vi "Elevator Loop.vi"() -> ()   [LabVIEW 2017]
uses:
  <vilib>/Rock Robotics/WPI/ThirdParty/Phoenix-LabVIEW/Motor Controller/Controls/CTRE_Phoenix_MotorControl_ControlMode.ctl
  <vilib>/Rock Robotics/WPI/ThirdParty/Sensors/navX/_TypeDefs/FRIC_navX_DeviceNumbersTypeDef.ctl
  Robot Global Data.vi
  <vilib>/Rock Robotics/WPI/Solenoid/Deprecated/WPI_SolenoidSetBool.vi
panel:
  out "Reverse Limit Closed?":bool
  out "Forward Limit Closed?":bool
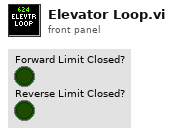
[diagram p1: front panel]
types:
  T1 = typedef "FRIC_navX_DeviceNumbersTypeDef.ctl" = enum16{"Dev0", "Dev1", "Dev2", "Dev3"}
  T2 = typedef "CTRE_Phoenix_MotorControl_ControlMode.ctl" = u16
  T3 = typedef "Dashboard Control Data.ctl" = cluster{"Drivetrain Settings Cluster":T4, "Intake Presets":T6, "Elevator Settings Cluster":T7, "Drivetrain Encoder Values":T9, "Auton Chooser":T10, "Auton Presets":cluster{"Start Position":dbl}, "Elevator Encoder Values":T11, "Pressure M":dbl, "Pressure B":dbl, "Zero All?":bool, "Enable Vision":bool}
  T4 = typedef "Drivetrain Settings Cluster.ctl" = cluster{"Gyro Steer PID Gains":T5, "Distance Drive PID Gains":T5, "Drive Tolerance":dbl, "Gyro Tolerance":dbl, "Gyro Output":dbl, "Distance Output":dbl, "Y Power Multiplier":dbl, "Turn Power Multiplier":dbl, "Creep Rate":dbl, "Encoder Reset":bool, "DT Mode Modifier":enum16{"None, Default", "Cube", "Square"}, "Left Encoder Tick Constant":dbl, "Right Encoder Tick Constant":dbl, "Shift Speed":dbl, "Zero Gyro":bool, "Y min":dbl, "Y max":dbl, "X min":dbl, "X max":dbl, "Finish Velocity":dbl, "Anti-tip peRcEnT":dbl}
  T5 = typedef "PID Gains Cluster.ctl" = cluster{"Proportional Gain":dbl, "Integral Time":dbl, "Derivative Time":dbl}
  T6 = typedef "Intake Presets.ctl" = cluster{"Idle Angle":dbl, "Mid Angle":dbl, "Low Angle":dbl, "Outtake Power":dbl, "Intake Power":dbl, "Unstuck":dbl, "Angle Tolerance":dbl, "Max Angle":dbl, "Max Current":dbl, "Current Trip Time":dbl, "Reset Encoder?":bool, "Encoder Scale":dbl, "PID gains":cluster{"proportional gain (Kc)":dbl, "integral time (Ti, min)":dbl, "derivative time (Td, min)":dbl}, "output range":cluster{"output high":dbl, "output low":dbl}, "IR Constant Pull Rate":dbl}
  T7 = typedef "Elevator Settings Cluster.ctl" = cluster{"Ground Height":dbl, "Switch Height":dbl, "Scale High Height ":dbl, "Scale Low Height":dbl, "Elevator PID Gains":T8, "Elevator Tolerance":dbl, "Reset Encoders":bool, "Encoder Scale":dbl, "Max Height":dbl, "Mid Height":dbl, "output range":cluster{"output high":dbl, "output low":dbl}, "Slow Down Tolerance":dbl, "Tick Constant":dbl, "Tip Constant":dbl, "Slow Down Multiplier":dbl, "Almost Tip Constant":dbl, "Bottom Trip Offset":dbl}
  T8 = typedef "PID Gains.ctl" = cluster{"proportional gain (Kc)":dbl, "integral time (Ti, min)":dbl, "derivative time (Td, min)":dbl}
  T9 = typedef "DT Encoder Values.ctl" = cluster{"Left Encoder":cluster{"Distance":dbl, "Speed":dbl, "Tick":dbl}, "Right Encoder":cluster{"Distance":dbl, "Speed":dbl, "Tick":dbl}}
  T10 = typedef "Auton Chooser.ctl" = cluster{"Left":bool, "Center":bool, "Right":bool, "Scale":bool, "Both":bool, "Switch":bool, "Test":bool, "No Script":bool}
  T11 = typedef "Elevator Encoder Values.ctl" = cluster{"Encoder Values":cluster{"Distance":dbl, "Speed":dbl, "Tick":dbl}}
  T12 = typedef "Dashboard Status Data.ctl" = cluster{"Elevator Status Cluster":T13, "Drivetrain Status Cluster":T16, "Intake Status Cluster":T18, "Climb Status Cluster":T21, "Intake PDP Info":T22, "Auton Command Cluster":T23, "Pressure ":dbl, "Auton Field Index":i32, "Auton File Index":i32, "Auton Side Index":i32, "Auton Side":string, "Field Config":string, "Robot Info":T24, "Auton Queue Index ":i32, "IMU Pitch Zero":dbl, "IMU Roll Zero":dbl, "IMU Yaw Zero":dbl}
  T13 = typedef "Elevator Status Cluster.ctl" = cluster{"Finished":bool, "Elevator Power":dbl, "Elevator State":T14, "Elevator Mode":T15, "Elevator Height":dbl, "At Bottom?":bool, "At Top?":bool, "Scale high?":bool, "PID Output":dbl, "2nd Gear":bool}
  T14 = typedef "Elevator State.ctl" = enum16{"Idle", "Ground", "Mid", "Scale", "Switch"}
  T15 = typedef "Elevator Mode.ctl" = enum16{"Semi Auto", "Manual", "Auto"}
  T16 = typedef "Drivetrain Status Cluster.ctl" = cluster{"Throttle (Y)":dbl, "Steer (X)":dbl, "Drivetrain Mode":T17, "Brake?":bool, "Distance Drive Complete?":bool, "PID Drive Complete?":bool, "Creep Mode?":bool, "Gyro Steer Complete?":bool, "Gyro":dbl, "Heading Target":dbl, "Distance Target":dbl, "2nd Gear":bool, "Drivetrain Encoder Values":T9}
  T17 = typedef "Drivetrain Mode.ctl" = enum16{"Manual", "Gyro Steer", "PID Drive", "Distance Drive", "Autonomous"}
  T18 = typedef "Intake Status Cluster.ctl" = cluster{"Intake Mode":T19, "Intake States":T20, "Intake Current Angle":dbl, "Cube In Posession?":bool, "Intake Wrist Up?":bool, "Right Roller Power":dbl, "Angle Power":dbl, "Left Roller Power":dbl}
  T19 = typedef "Intake Mode.ctl" = enum16{"Auto", "Semi Auto", "Manual"}
  T20 = typedef "Intake States.ctl" = enum16{"Zero", "Override Angle", "Idle", "Drop Mid", "Drop Low", "Outtake", "Intake"}
  T21 = typedef "Climb Status Cluster.ctl" = cluster{"Climb":bool, "Time Remaining":dbl, "Button Pressed":bool}
  T22 = typedef "Intake PDP Info.ctl" = cluster{"Voltage Percent Output":dbl, "Output Voltage":dbl, "Bus Voltage":dbl, "Device ID":dbl, "Output Current":dbl, "Sensor Velocity":dbl, "Sensor Position":dbl, "Pulse Width Position":dbl, "Pulse Width Velocity":dbl, "Temperature":dbl, "Inverted?":bool}
  T23 = typedef "Auton Command Cluster.ctl" = cluster{"commandID":dbl, "headingTarget":dbl, "async":dbl, "elevatorCommand":dbl, "intakeMode":dbl, "maxTime":dbl, "ySpeed":dbl, "zeroGyro":dbl, "intakeCommand":dbl, "distanceTarget":dbl, "xSpeed":dbl, "elevatorMode":dbl, "scaleHigh":dbl, "rollerSpeed":dbl, "intakeAngle":dbl, "manualOpen":dbl, "secondGear":dbl, "elevatorPower":dbl, "waitFor":dbl, "overrideAngle":dbl}
  T24 = typedef "Robot Info.ctl" = cluster{"FMS":bool, "Switch and Scale Sides":string, "Event Name":string, "Alliance":T25, "Position":T26, "Match Number":u16, "Robot Mode":T27, "Match Time(s)":sgl}
  T25 = typedef "WPI_DriverStationAllianceInfo.ctl" = enum16{"Red", "Blue", "Invalid"}
  T26 = typedef "WPI_DriverStationPositionInfo.ctl" = enum16{"1", "2", "3"}
  T27 = typedef "WPI_DriverStationRobotMode2.ctl" = enum16{"Autonomous Disabled", "Autonomous Enabled", "Teleop Disabled", "Teleop Enabled", "Disconnected", "Finish", "Test Disabled", "Test Enabled", "Emergency Stopped"}
  T28 = typedef "Elevator Command Cluster.ctl" = cluster{"Elevator Mode":T15, "Elevator State":T14, "Manual Speed":dbl, "Reset Encoders":bool, "High?":bool, "Climb?":bool, "Gear 2?":bool}
  T29 = typedef "WPI_SolenoidDevRef.ctl" = cluster{"DevStatus":errorcluster, "Pneumatics Control Module":u8, "Forward Solenoid Channel":T30, "Reverse Solenoid Channel":T30}
  T30 = typedef "WPI_SolenoidChannel.ctl" = enum8{"Solenoid 0", "Solenoid 1", "Solenoid 2", "Solenoid 3", "Solenoid 4", "Solenoid 5", "Solenoid 6", "Solenoid 7", "Invalid"}
  T31 = cluster{"Yaw":dbl, "Roll":dbl, "Pitch":dbl, "Heading":dbl, "Fused Heading":dbl}
  T32 = typedef "WPI_SwitchDevRef.ctl" = cluster{"DevStatus":errorcluster, "DIO Channel":T33, "CntIndex":T34, "Normally Closed":bool}
  T33 = typedef "FPGA_DIOChannel.ctl" = enum8{"DIO 0", "DIO 1", "DIO 2", "DIO 3", "DIO 4", "DIO 5", "DIO 6", "DIO 7", "DIO 8", "DIO 9", "DIO MXP 0", "DIO MXP 1", "DIO MXP 2", "DIO MXP 3", "DIO MXP 4", "DIO MXP 5", "DIO MXP 6", "DIO MXP 7", "DIO MXP 8", "DIO MXP 9", "DIO MXP 10", "DIO MXP 11", "DIO MXP 12", "DIO MXP 13", "DIO MXP 14", "DIO MXP 15", "SPI Port CS1", "SPI Port CS2", "SPI Port CS3", "SPI Port MISO", "SPI Port MOSI", "Invalid"}
  T34 = typedef "FPGA_CounterCtrSystemIndex.ctl" = enum8{"Ctr 0", "Ctr 1", "Ctr 2", "Ctr 3", "Ctr 4", "Ctr 5", "Ctr 6", "Ctr 7", "Invalid"}
  T35 = typedef "WPI_MotorControlDeviceRef.ctl" = cluster{"DeviceStatus":errorcluster, "Type":T36, "PWM":cluster{"PWM Channel":T37, "DeadBand":T38}, "CAN":cluster{"Device Number":u8, "SetOutput VI Ref":variant, "GetOutput VI Ref":variant, "Enable VI Ref":variant, "Disable VI Ref":variant, "Data":variant}, "Invert":bool, "DIO PWM":cluster{"PWM \"Enable\" Channel":T37, "DIOChannel":T33, "PWM Rate":dbl}}
  T36 = typedef "WPI_MotorControlType.ctl" = enum16{"PWM", "CAN", "DIO PWM"}
  T37 = typedef "FPGA_DIOPWMChannel.ctl" = enum8{"PWM 0", "PWM 1", "PWM 2", "PWM 3", "PWM 4", "PWM 5", "PWM 6", "PWM 7", "PWM 8", "PWM 9", "PWM MXP 0", "PWM MXP 1", "PWM MXP 2", "PWM MXP 3", "PWM MXP 4", "PWM MXP 5", "PWM MXP 6", "PWM MXP 7", "PWM MXP 8", "PWM MXP 9", "Invalid"}
  T38 = typedef "WPI_PWMDeadband.ctl" = cluster{"Name":string, "maxPositivePwm":i32, "minPositivePwm":i32, "centerPwm":i32, "maxNegativePwm":i32, "minNegativePwm":i32, "angularRange":u16}
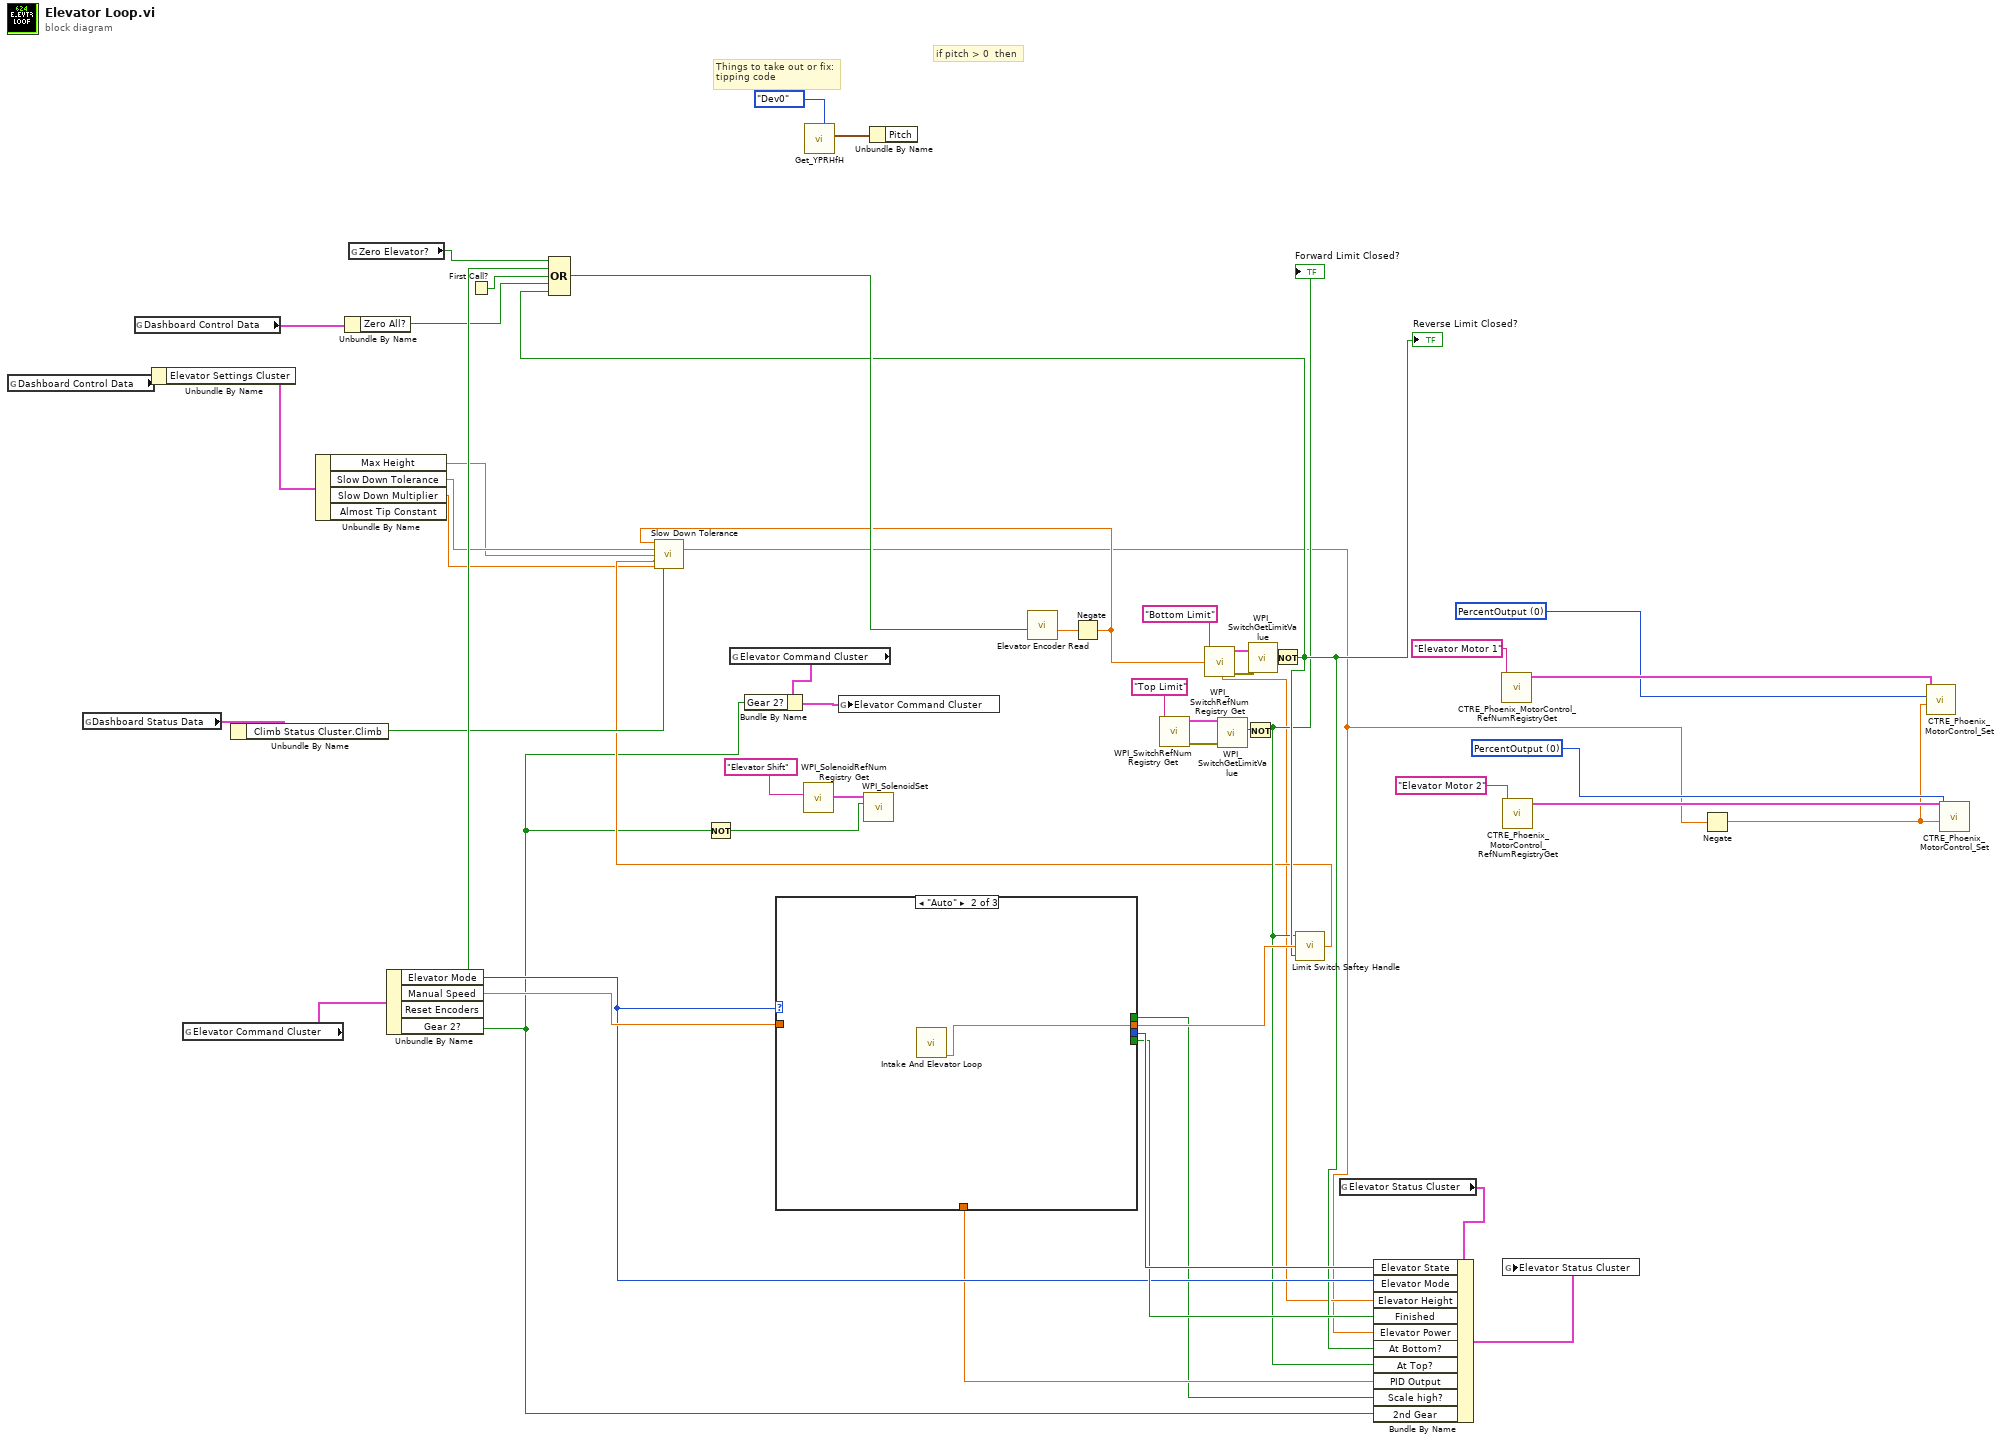
[diagram p0: block diagram]
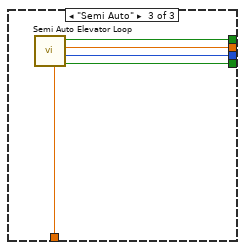
[diagram p3: hidden frame]
diagram:
  w37 = T2 0 items=["PercentOutput"=0, "Position"=1, "Velocity"=2, "Current"=3, "Follower"=5, "MotionProfile"=6, "MotionMagic"=7, "MotionMagicArc"=8, "MotionProfileArc"=10, "Disabled"=15] ("Control Mode")
  w36 = T2 0 items=["PercentOutput"=0, "Position"=1, "Velocity"=2, "Current"=3, "Follower"=5, "MotionProfile"=6, "MotionMagic"=7, "MotionMagicArc"=8, "MotionProfileArc"=10, "Disabled"=15] ("Control Mode")
  # "if pitch > 0  then"
  # "Things to take out or fix:\ntipping code"
  n1 = global read "Robot Global Data.vi" "Dashboard Control Data"() -> (w46:T3)
  n2 = global read "Robot Global Data.vi" "Dashboard Status Data"() -> (w31:T12)
  n3 = global read "Robot Global Data.vi" "Dashboard Control Data"() -> (w6:T3)
  n4 = Unbundle By Name(w46) -> ("Elevator Settings Cluster"=w45:T7)
  n5 = global read "Robot Global Data.vi" "Elevator Command Cluster"() -> (w42:T28)
  n6 = Unbundle By Name(w31) -> ("Climb Status Cluster.Climb"=w28:bool)
  n7 = Unbundle By Name(w45) -> ("Max Height"=w29:dbl, "Slow Down Tolerance"=w30:dbl, "Slow Down Multiplier"=w13:dbl)  [unwired: 1 out]
  n8 = Unbundle By Name(w6) -> ("Zero All?"=w5:bool)
  n9 = global read "Robot Global Data.vi" "Zero Elevator?"() -> (w44:bool)
  n10 = Unbundle By Name(w42) -> ("Elevator Mode"=w35:T15, "Manual Speed"=w41:dbl, "Reset Encoders"=w32:bool, "Gear 2?"=w1:bool)
  n11 = First Call?() -> (First Call?: T/F=w43:bool)
  n12 = Not(x=w1) -> (.not. x?=w2:bool)
  n13 = global read "Robot Global Data.vi" "Elevator Command Cluster"() -> (w11:T28)
  n14 = Bundle By Name(cluster=w11, "Gear 2?"=w1) -> (w12:T28)
  n15 = case shown="\"Auto\"" w35 {
    tunnel: [w53 w54 w59] -> w38
    tunnel: w41 -> [w53 _ _]
    tunnel: [_ _ w58] -> w40
    tunnel: [_ _ w57] -> w39
    tunnel: [_ _ w56] -> w33
    tunnel: [_ _ w55] -> w34
    frame "Manual", Default {
    }
    frame "Auto" {
      n16 = call "Intake And Elevator Loop.vi"() -> ("Elevator Power"=w54:dbl)  [unwired: 11 in, 4 out]
    }
    frame "Semi Auto" {
      n17 = call "Semi Auto Elevator Loop.vi"() -> ("Finished?"=w57:bool, "Elevator State"=w58:T14, "Elevator Power"=w59:dbl, "High?"=w56:bool, "PID Output"=w55:dbl)  [unwired: 7 in]
    }
  }
  n18 = call <vilib>:"WPI_SolenoidRefNum Registry Get.vi"("refnum name"="Elevator Shift") -> ("SolenoidDevRef"=w9:T29)  [unwired: 9 in, 1 out]
  n19 = call <vilib>:"Get_YPRHfH.vi"("Device Number"=FRIC_navX_DeviceNumbersTypeDef."Dev0") -> ("YRPHfH"=w3:T31)  [unwired: 10 in]
  n20 = global write "Robot Global Data.vi" "Elevator Command Cluster"(w12) -> ()
  n21 = call-poly <vilib>:"WPI_SolenoidSet.vi"("Value"=w2, "SolenoidDevRef"=w9) -> ()  [unwired: 8 in, 2 out]
  n22 = Unbundle By Name(w3) -> ()  [unwired: 1 out]
  n23 = call <vilib>:"WPI_SwitchRefNum Registry Get.vi"("refnum name"="Top Limit") -> ("error out"=w25:errorcluster, "SwitchDevRef"=w24:T32)  [unwired: 9 in]
  n24 = call <vilib>:"WPI_SwitchRefNum Registry Get.vi"("refnum name"="Bottom Limit") -> ("error out"=w23:errorcluster, "SwitchDevRef"=w22:T32)  [unwired: 9 in]
  n25 = call <vilib>:"WPI_SwitchGetLimitValue.vi"("error in (no error)"=w25, "SwitchDevRef"=w24) -> ("Switch Pressed"=w18:bool)  [unwired: 7 in, 2 out]
  n26 = Not(x=w18) -> (.not. x?=w17:bool)
  "Forward Limit Closed?" <- w17
  n27 = call <vilib>:"WPI_SwitchGetLimitValue.vi"("error in (no error)"=w23, "SwitchDevRef"=w22) -> ("Switch Pressed"=w20:bool)  [unwired: 7 in, 2 out]
  n28 = Not(x=w20) -> (.not. x?=w19:bool)
  "Reverse Limit Closed?" <- w19
  n29 = Compound Arithmetic op=OR(w44, w32, w43, w5, w19) -> (w21:bool)
  n30 = call "Elevator Encoder Read.vi"("Reset?"=w21) -> ("Height"=w15:dbl)  [unwired: 10 in]
  n31 = Negate(x=w15) -> (-x=w14:dbl)
  n32 = call "Limit Switch Saftey Handle.vi"("Lower Limit"=w19, "Motor In"=w38, "Upper Limit"=w17) -> ("Motor Out"=w16:dbl)
  n33 = call "Slow Down Tolerance.vi"("Current Height"=w14, "Slow Down Tolerance"=w30, "Max Height"=w29, "Elevator Power"=w16, "Slow Down Multiplier"=w13, "Climb"=w28) -> ("Motor Out"=w8:dbl)  [unwired: 9 in]
  n34 = global read "Robot Global Data.vi" "Elevator Status Cluster"() -> (w48:T13)
  n35 = Bundle By Name(cluster=w48, "Elevator State"=w40, "Elevator Mode"=w35, "Elevator Height"=w14, "Finished"=w39, "Elevator Power"=w8, "At Bottom?"=w19, "At Top?"=w17, "PID Output"=w34, "Scale high?"=w33, "2nd Gear"=w1) -> (w47:T13)
  n36 = call <vilib>:"CTRE_Phoenix_MotorControl_RefNumRegistryGet.vi"("refnum name"="Elevator Motor 1") -> ("PhoenixMotorControlDevRef"=w52:T35)  [unwired: 9 in, 1 out]
  n37 = call <vilib>:"CTRE_Phoenix_MotorControl_RefNumRegistryGet.vi"("refnum name"="Elevator Motor 2") -> ("PhoenixMotorControlDevRef"=w50:T35)  [unwired: 9 in, 1 out]
  n38 = global write "Robot Global Data.vi" "Elevator Status Cluster"(w47) -> ()
  n39 = Negate(x=w8) -> (-x=w7:dbl)
  n40 = call <vilib>:"CTRE_Phoenix_MotorControl_Set.vi"("Output"=w7, "Control Mode"=w36, "PhoenixMotorControlDevRef"=w52) -> ()  [unwired: 7 in, 2 out]
  n41 = call <vilib>:"CTRE_Phoenix_MotorControl_Set.vi"("Output"=w7, "Control Mode"=w37, "PhoenixMotorControlDevRef"=w50) -> ()  [unwired: 7 in, 2 out]
